vi "Report Avg Power.vi"(8 "error in (no error)":errorcluster, 11 "ReturnPwr":dbl) -> (0 "error out":errorcluster)   [LabVIEW 2013, in "QCAWLAN_DLL.lvlib"]
doc: "QCA_DLL_Export void ReportAvgPower(double ReturnPwr);"
uses:
  QCAWLAN_DLL.lvlib
  QCAWLAN_DLL.dll
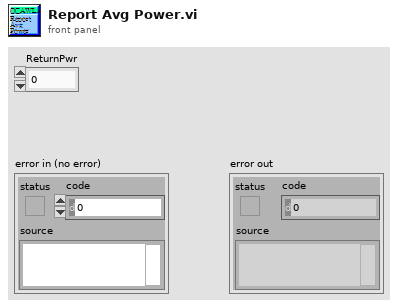
[diagram p1: front panel]
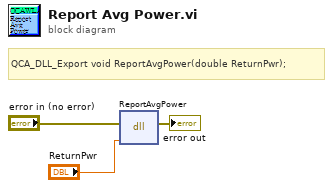
[diagram p0: block diagram]
diagram:
  # "QCA_DLL_Export void ReportAvgPower(double ReturnPwr);"
  n1 = dll-call lib="C:/Connectivity Client - MIMO/PlugIn/QCAWLAN_DLL.*" fn="ReportAvgPower"(error in="error in (no error)", "ReturnPwr"="ReturnPwr") -> (error out=→"error out":errorcluster)  [unwired: 4 in, 1 out]
